vi "rqcBob Key Distribution (Low Level Example).vi"() -> ()   [LabVIEW 2018]
uses:
  FPGA/rqcBob/Custom Controls/rqcBob Trigger Type.ctl
  Custom Controls/rqcBob States.ctl
  Shared/Shared FPGA Lib/Shared Logic/Custom Controls/rqc Random Generator.parameters.ctl
  Shared/Shared FPGA Lib/Shared Logic/Custom Controls/rqc Random Generator.value type.ctl
  FPGA/rqcBob/Custom Controls/rqcBob Window Config.ctl
  FPGA/rqcBob/Custom Controls/rqcBob Modulator Config.ctl
  FPGA/rqcBob/Custom Controls/Pulse Train/rqcBob Pulse Train Config.ctl
  FPGA/rqcBob/Custom Controls/Pulse Train/rqcBob Pulse Train.Generation Mode.ctl
  FPGA/rqcBob/Custom Controls/Pulse Train/rqcBob Pulse Train.First Pulse Delay Mode.ctl
  Shared/Shared Host Lib/rqc ServiceNET/Custom Controls/rqc ServiceNET command.ctl
  Shared/Shared Host Lib/rqc ServiceNET/Bob/Custom Controls/rqcBob ServiceNET control.ctl
  <vilib>/FPGAPlugInAG/PCIe-7820R/niLvFpga_Open_PCIe-7820R.vi
  <vilib>/rvi/interface/common/dynamic/niFpgaDynamicAddResources.vi
  Low Level API/Configuration/Photon Detector/Set PD window/rqcBob Configure SPD Detection Window (2PD).vi
  Shared/Shared Host Lib/rqc ServiceNET/Bob/rqcBob Send Data/rqcBob ServiceNET Send Data U32.vi
  <vilib>/FPGAPlugInAG/Dynamic/niLvFpga_Close_Dynamic.vi
  <vilib>/rvi/interface/nirviOpenFPGA/nirviOpenFPGA.xnode
  FPGA Bitfiles/rqcBob (FPGA) 7820 v 4.0.0.lvbitx
  <vilib>/rvi/interface/nirviCloseFPGA/nirviCloseFPGA.xnode
panel:
  out "Bob's Key:":string="010100110101111110011011110000111111100101101001011100110010001011010011011001010000111101100001111011001111110010010110111100010001111011001000011001001101011000010111001010101110111010010000110011001101101100100101111100001111001011011110000010010101011001111010111001111100111110100100111011110001110101001100010011010001011011101010101000100011010101011010010001111110100010011010011001101101101000001100010110011001101001010101011000110010101100111101110101110011110100101100100001100100001101100001110010011000001101111001111110101101001010000110011100000011111101100010010100111000101011100110111010011100100000110000100110111101100000011011010011110000111011110111001101110001101011100111000010001001011000101100001110011001000100110101110010100000011011000001100111000101000100001110001001001011101100101101111000011101000111001110111000000101101000101011110101001101000001001000010011001010000011111111010010010001111011111001110001010100000010001000000101000000100101011010110100010111110111011110001100101010110010011101001010001100100000110000001111110101000001010000110001000011101110100110001000001100010101001000"
  in  "Modulator shift":fxp<+,4,4>=2.0
  in  "Check D2":u8=6
  in  "Random\nOn/Off":bool=TRUE
  in  "Pi Voltage":u16=140
  in  "2-Random (Up)\n4-Random (Down)":bool
  in  "Train Number":u16=1000
  in  "Pulses in Train":u16=500
  in  "Train Period":u16=4000
  in  "Open window":u16=2530
  out "Key length (s)":i32=2253
  out "Incorrect Alice's data":bool
  out "Total pulses expected:":u32=500000
  in  "Data shift":u8=3
  out "Current States":dbl=13.0
  out "error out":errorcluster
  out "Connected to Alice":bool
  in  "Stop":bool
  in  "Check D1":u8=24
  in  "Port:":u16=5020
  in  "Alice's IP address":string="192.168.0.175"
  # "BOB"
  # "FPGA settings:"
  # "LAN settings:"
  # "Key distillation details:"
  # "Data exchange details:"
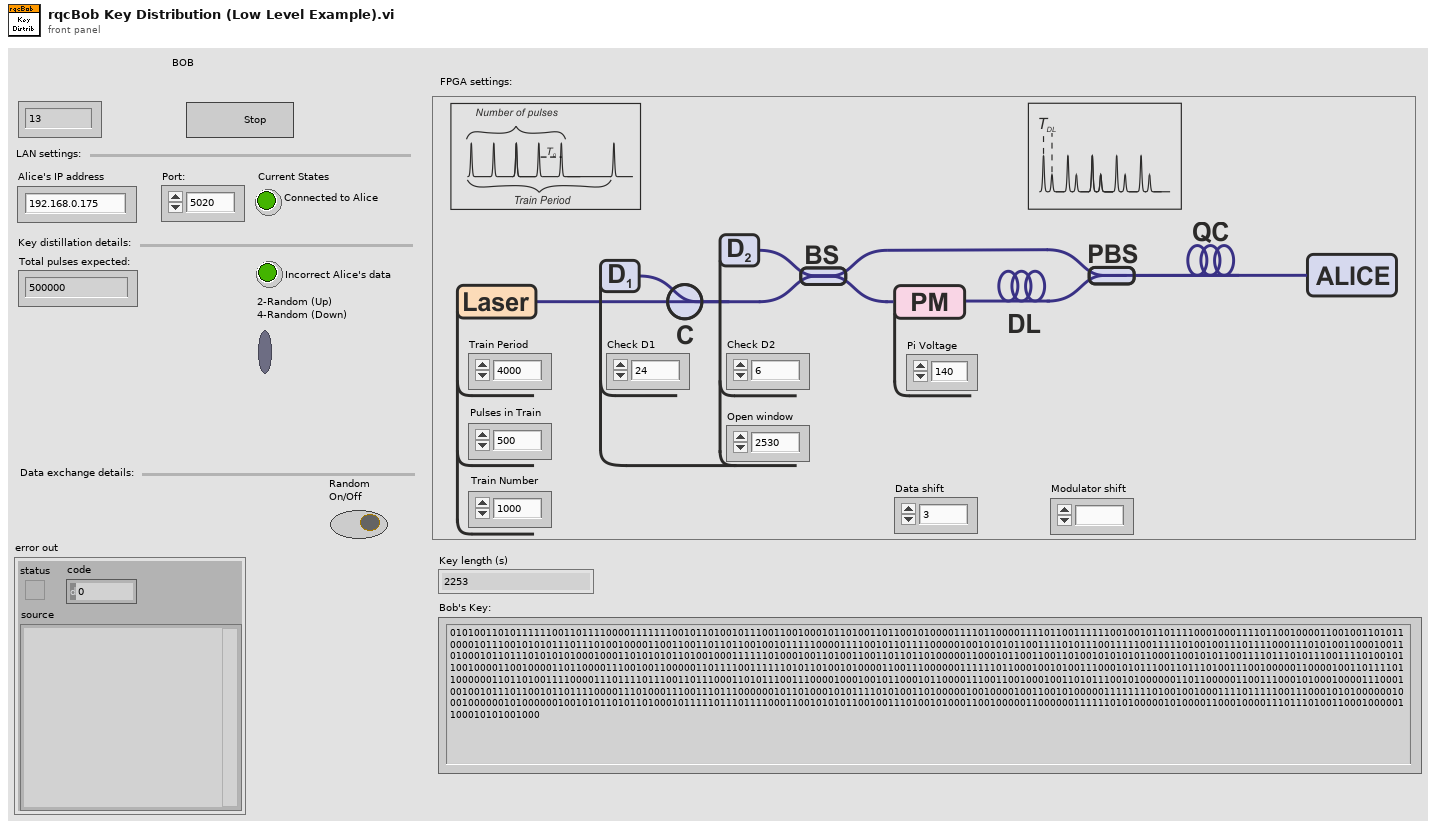
[diagram p1: front panel]
types:
  T1 = typedef "rqcBob States.ctl" = enum16{"HW.configure", "HW.sendTrigger", "HW.initiate", "HW.measure", "HW.stop", "NET.create", "NET.connect", "NET.sendCommand", "NET.readCommand", "NET.readData", "NET.close", "App.HandleEvent", "App.HandleError", "App.Stop"}
  T2 = typedef "rqcBob Trigger Type.ctl" = enum16{"software", "immediate", "DIO"}
  T3 = typedef "rqcBob Pulse Train Config.ctl" = cluster{"period":u16, "num of pulses":u16, "mode":T4, "num of trains":u16, "first pulse delay mode":T5, "first pulse delay":u16}
  T4 = typedef "rqcBob Pulse Train.Generation Mode.ctl" = enum8{"single train", "train sequence.single", "train sequence.wait for trigger", "continuous"}
  T5 = typedef "rqcBob Pulse Train.First Pulse Delay Mode.ctl" = enum8{"none", "every train", "first train"}
  T6 = typedef "rqcBob Modulator Config.ctl" = cluster{"modulator.start":u16, "modulator.stop":u16}
  T7 = typedef "rqcBob Window Config.ctl" = cluster{"window.open":u16, "window.close":u16}
  T8 = typedef "rqc Random Generator.parameters.ctl" = cluster{"value type":T9, "constant":u16, "num of levels":u16, "levels values":u16[]}
  T9 = typedef "rqc Random Generator.value type.ctl" = enum16{"random value", "constant"}
  T10 = typedef "rqc ServiceNET command.ctl" = enum8{"NONE", "READY", "START", "PING", "SEND KEY", "WRITE KEY", "WRITE AND SAVE KEY"}
  T11 = typedef "rqcBob ServiceNET control.ctl" = cluster{"connection ID":refnum<k5>, "connected?":bool, "Alice's IP address":string, "port":u16}
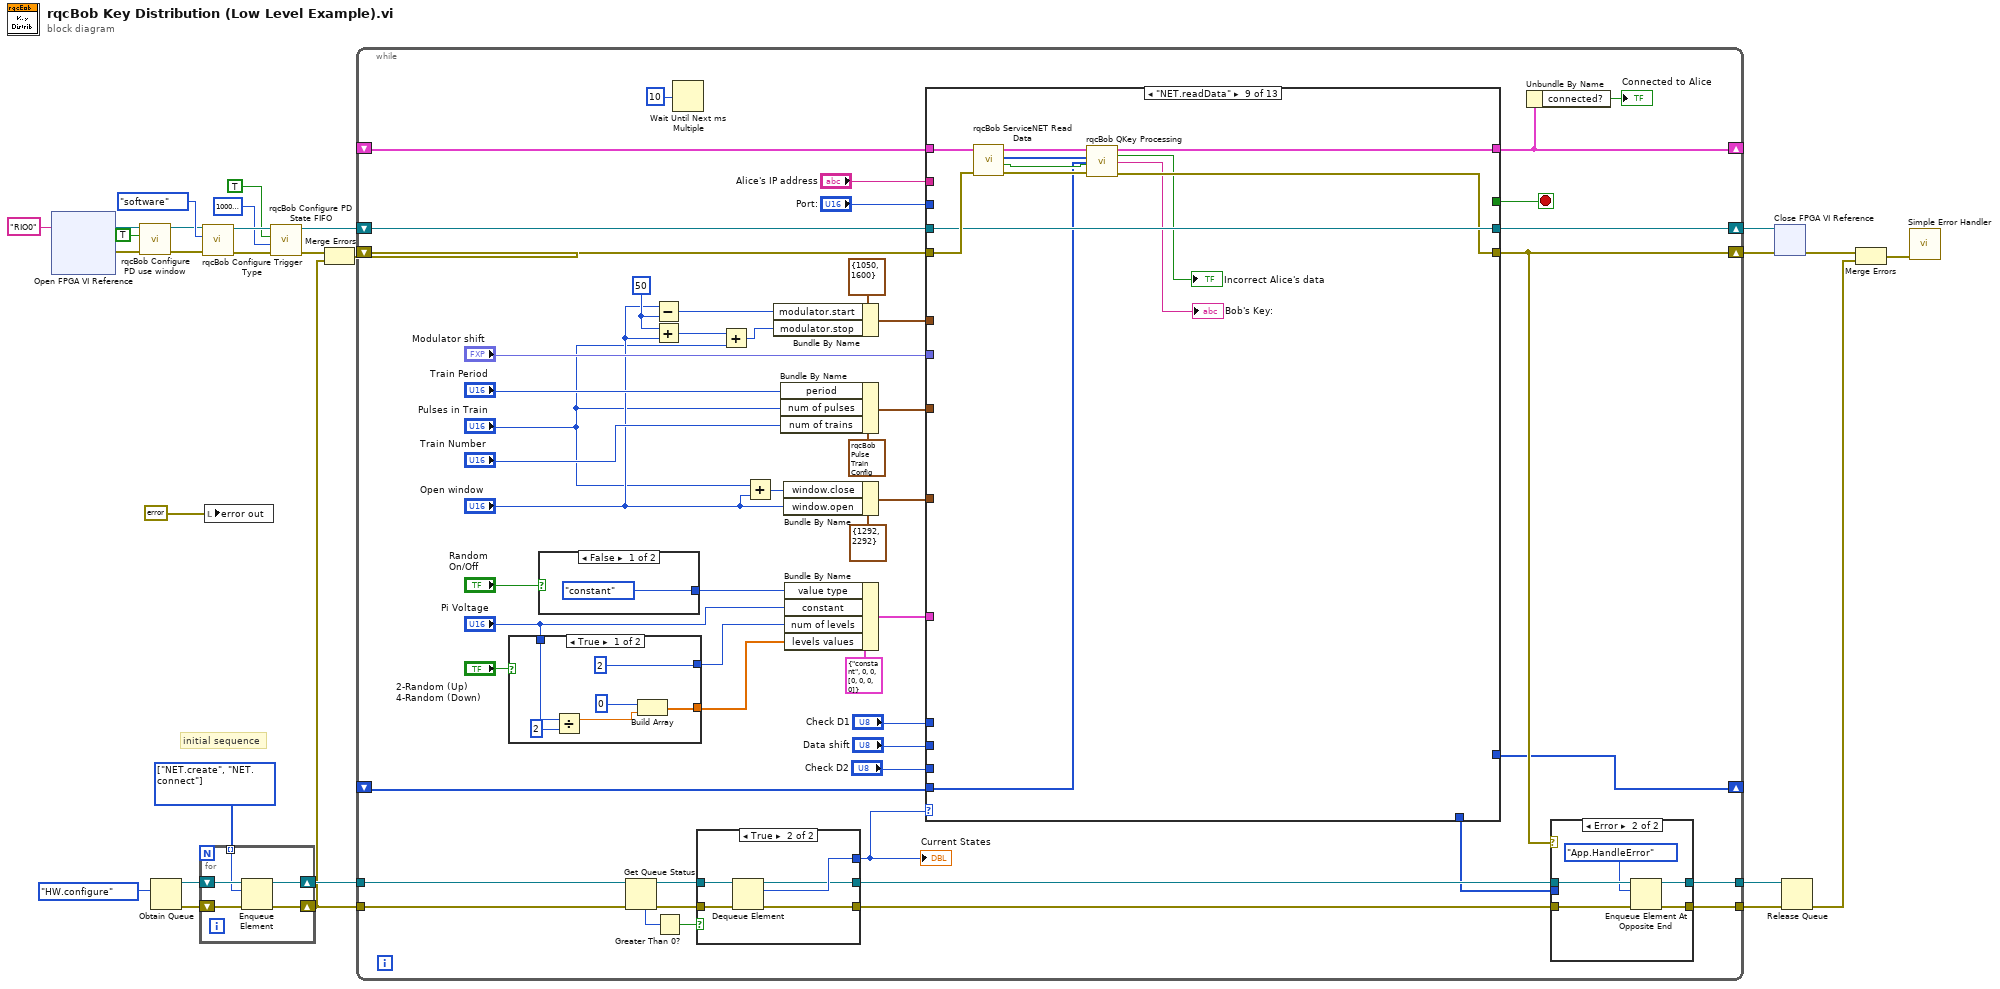
[diagram p0: block diagram]
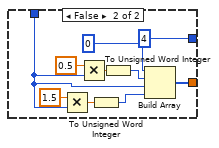
[diagram p2: hidden frame]
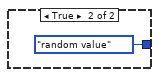
[diagram p3: hidden frame]
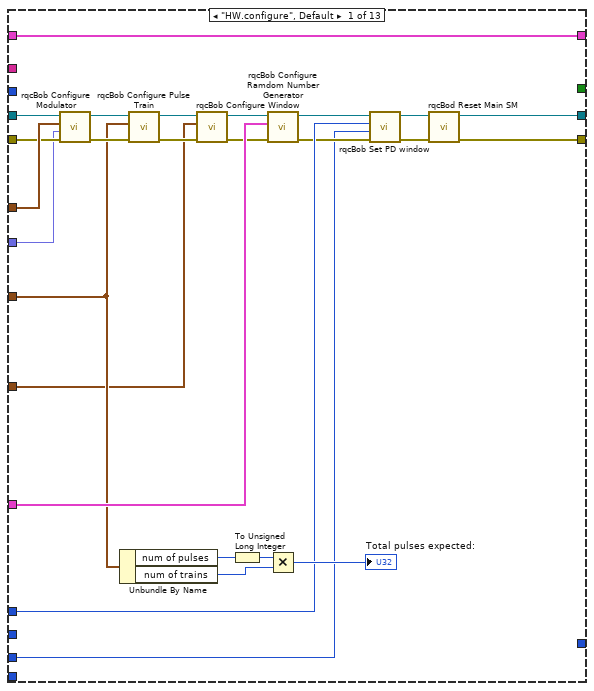
[diagram p4: hidden frame]
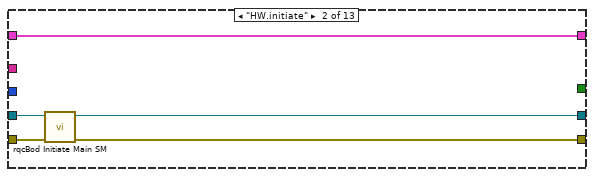
[diagram p5: hidden frame]
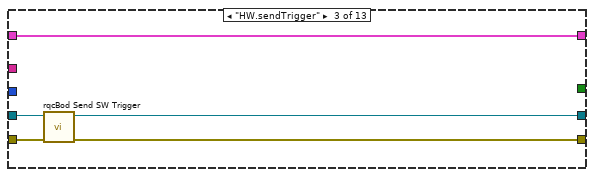
[diagram p6: hidden frame]
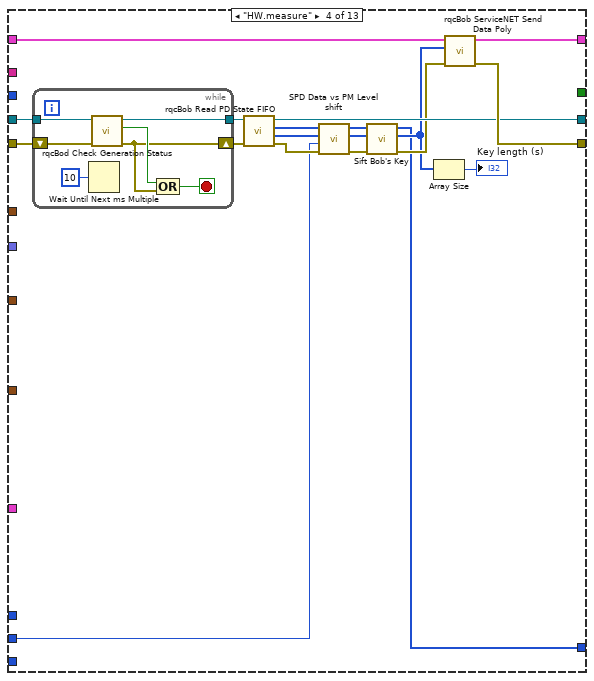
[diagram p7: hidden frame]
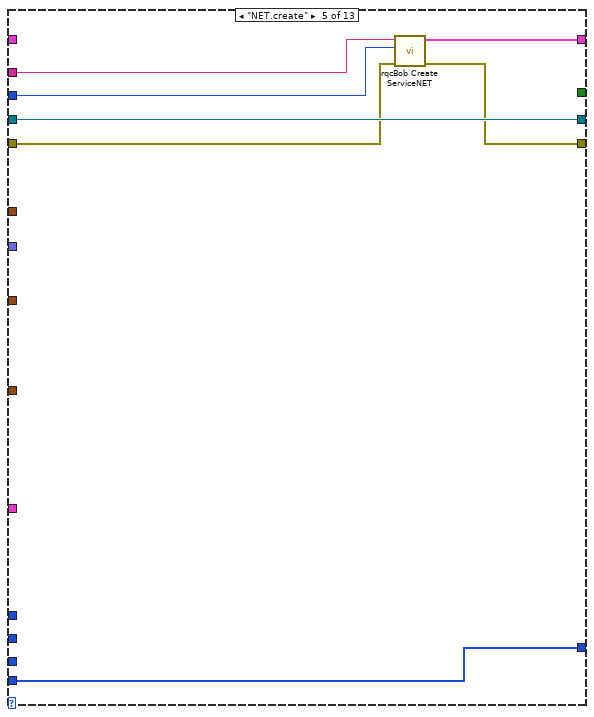
[diagram p8: hidden frame]
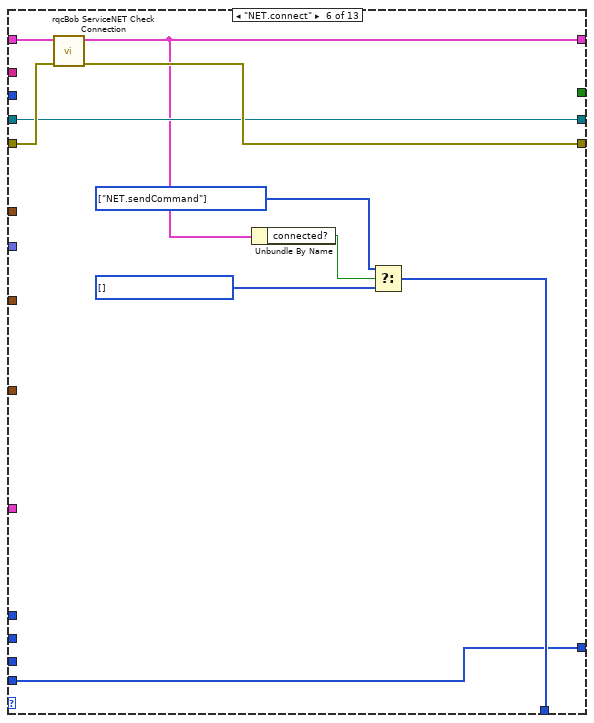
[diagram p9: hidden frame]
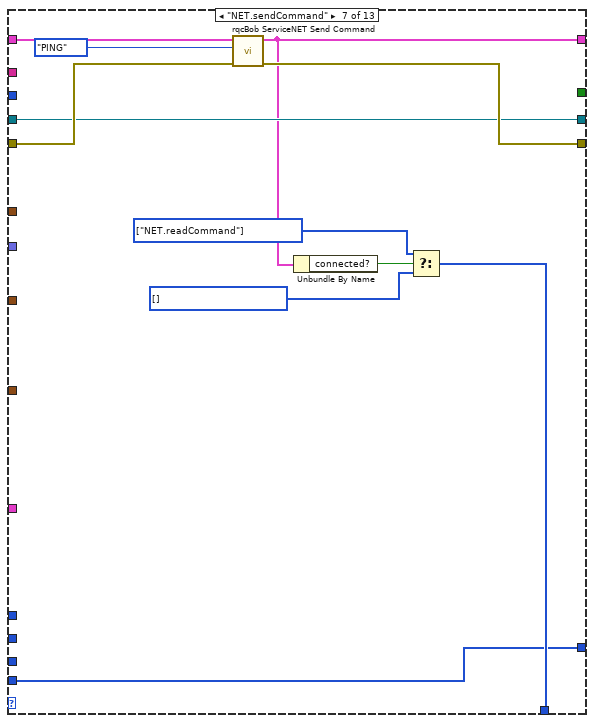
[diagram p10: hidden frame]
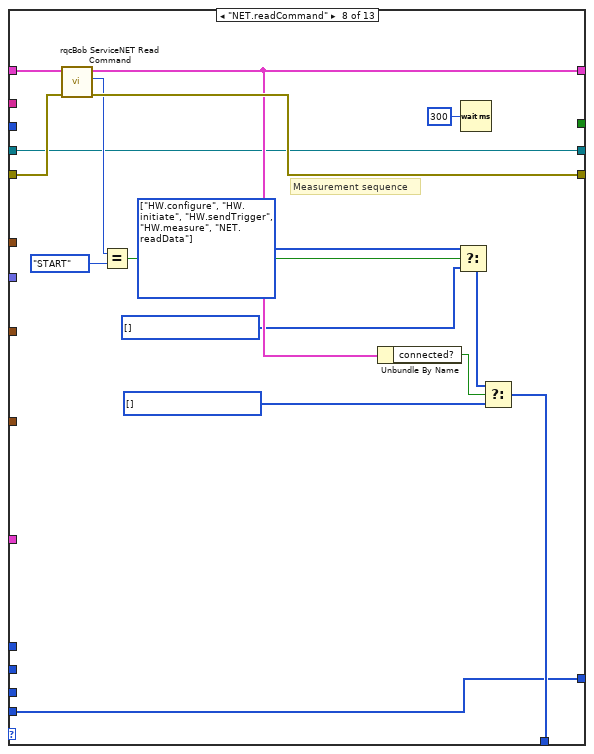
[diagram p11: hidden frame]
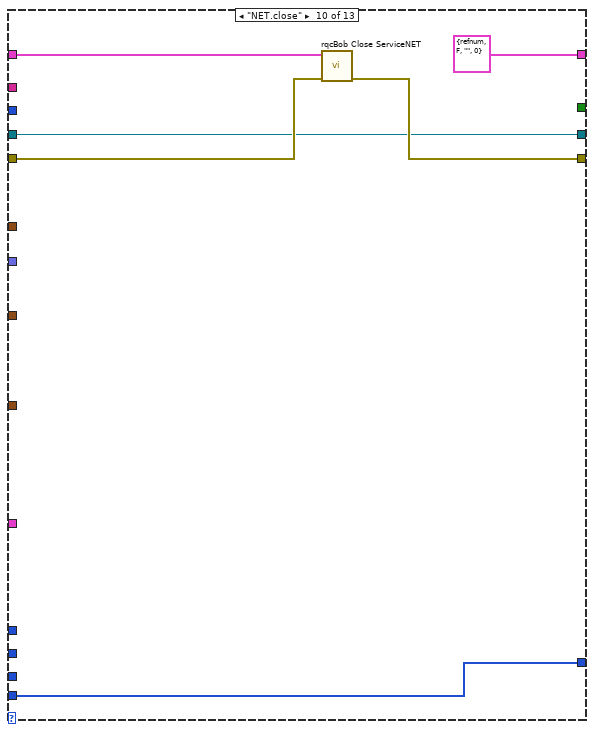
[diagram p12: hidden frame]
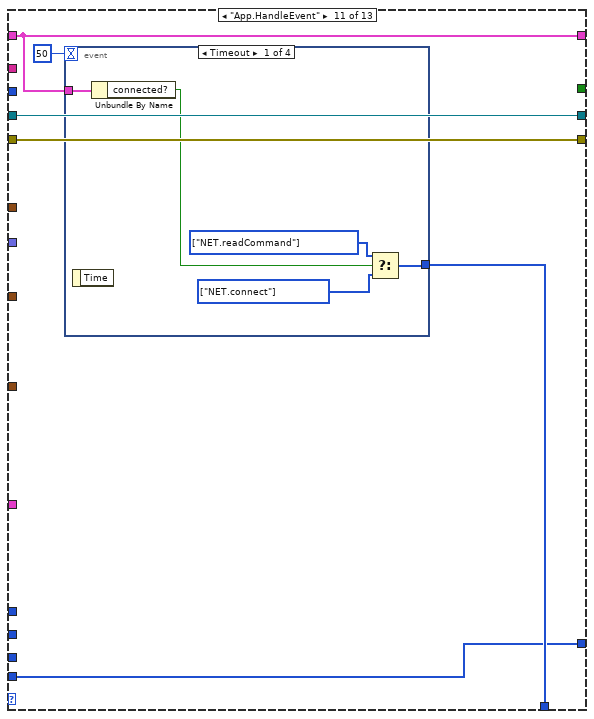
[diagram p13: hidden frame]
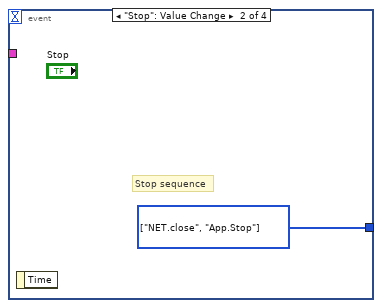
[diagram p14: hidden frame]
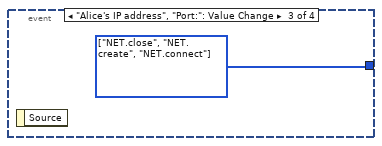
[diagram p15: hidden frame]
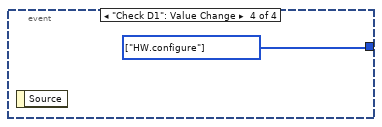
[diagram p16: hidden frame]
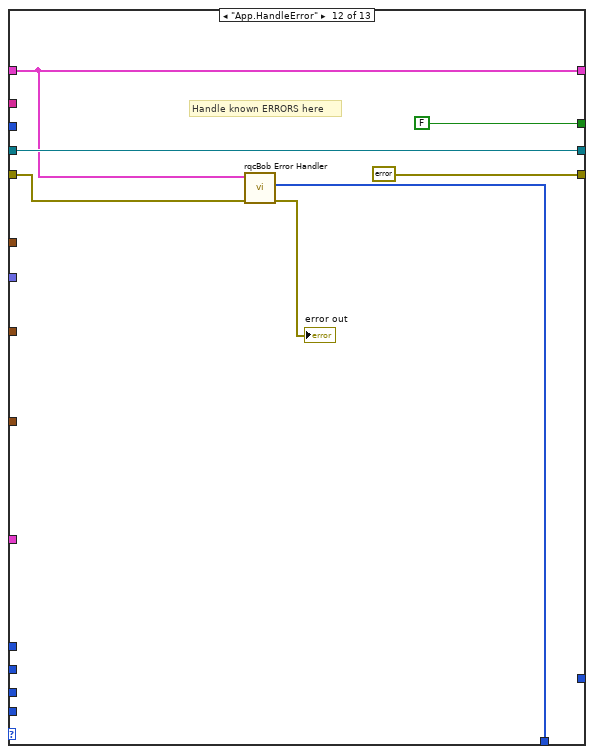
[diagram p17: hidden frame]
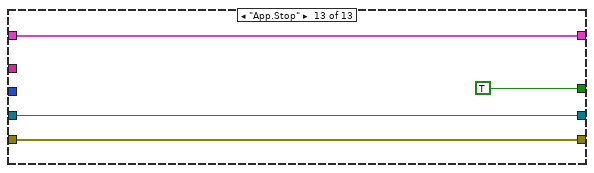
[diagram p18: hidden frame]
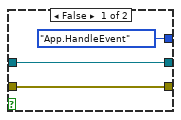
[diagram p19: hidden frame]
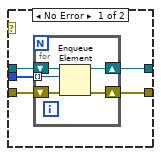
[diagram p20: hidden frame]
diagram:
  w21 = T1[] [enum."NET.create", enum."NET.connect"] items=["HW.configure", "HW.sendTrigger", "HW.initiate", "HW.measure", "HW.stop", "NET.create", "NET.connect", "NET.sendCommand", "NET.readCommand", "NET.readData", "NET.close", "App.HandleEvent", "App.HandleError", "App.Stop"]
  # "initial sequence"
  n1 = xnode "Open FPGA VI Reference"("resource name"="RIO0") -> ("FPGA VI Reference Out"=w5:refnum<k20>, "error out"=w3:errorcluster)  [unwired: 1 in]
  n2 = call "rqcBob Configure PD use window.vi"("error in"=w3, "PD.use window"=TRUE, "FPGA reference in"=w5) -> ("error out"=w2:errorcluster, "FPGA reference out"=w4:refnum<k20>)  [unwired: 7 in]
  n3 = Obtain Queue(element data type=rqcBob_States."HW.configure" ("rqcBob States")) -> (queue out=w26:refnum<queue>, error out=w25:errorcluster)  [unwired: 4 in, 1 out]
  n4 = for {
    tunnel: w21 -> [w29] mode=indexing
    shift-right: [w30] -> w23
    shift-left: w26 -> [w33]
    shift-right: [w31] -> w20
    shift-left: w25 -> [w32]
    n5 = Enqueue Element(queue=w33, element=w29, error in (no error)=w32) -> (queue out=w30:refnum<queue>, error out=w31:errorcluster)  [unwired: 1 in, 1 out]
  }
  n6 = call "rqcBob Configure Trigger Type.vi"("error in"=w2, "rqcBob Trigger Type"=rqcBob_Trigger_Type."software", "FPGA reference in"=w4) -> ("error out"=w8:errorcluster, "FPGA reference out"=w11:refnum<k20>)  [unwired: 7 in]
  n7 = local write "error out"(errorcluster {"status"=FALSE, "code"=0, "source"=""} ("error constant")) -> ()
  n8 = call "rqcBob Configure PD State FIFO.vi"("error in"=w8, "PD.state fifo depth"=u32 10000000 ("SPD.detect fifo depth"), "PD.state fifo write enable"=TRUE ("SPD.detect fifo write enable"), "FPGA reference in"=w11) -> ("error out"=w9:errorcluster, "FPGA reference out"=w10:refnum<k20>)  [unwired: 6 in]
  n9 = Merge Errors(w9, w20) -> (w24:errorcluster)
  n10 = while {
    shift-right: [w68] -> w19
    shift-left: w24 -> [w79]
    shift-right: [w69] -> w18
    shift-left: w10 -> [w66]
    tunnel: w23 -> [w77]
    tunnel: w20 -> [w76]
    tunnel: [w71] -> w17
    tunnel: [w70] -> w16
    shift-right: [w62] -> _
    shift-left: _ -> [w63]
    shift-right: [w58] -> _
    shift-left: _ -> [w57]
    stop <- w67 stop-if-true
    w49 = 50
    n11 = case shown="True" "2-Random (Up)\n4-Random (Down)" {
      tunnel: [w91 w92] -> w41
      tunnel: [u16 2 ("pm.DAC num of levels") u16 4 ("pm.DAC num of levels")] -> w40
      tunnel: "Pi Voltage" -> [w88 w93]
      frame True {
        n12 = Divide(x=w88, y=u16 2) -> (x/y=w87:dbl)
        n13 = Build Array(u16 0, w87) -> (w91:dbl[])
      }
      frame False {
        n14 = Multiply(x=1.5, y=w93) -> (x*y=w98:dbl)
        n15 = Multiply(x=0.5, y=w93) -> (x*y=w100:dbl)
        n16 = To Unsigned Word Integer(number=w98) -> (unsigned 16bit integer=w95:u16)
        n17 = To Unsigned Word Integer(number=w100) -> (unsigned 16bit integer=w96:u16)
        n18 = Build Array(u16 0, w96, w93, w95) -> (w92:u16[])
      }
    }
    n19 = case shown="False" "Random\nOn/Off" {
      tunnel: [rqc_Random_Generator.value_type."constant" ("value type") rqc_Random_Generator.value_type."random value" ("value type")] -> w42
      frame False {
      }
      frame True {
      }
    }
    n20 = Get Queue Status(queue=w77, error in (no error)=w76) -> (queue out=w73:refnum<queue>, error out=w72:errorcluster, # elements in queue=w75:i32)  [unwired: 1 in, 5 out]
    n21 = Subtract(x="Open window", y=w49) -> (x-y=w46:i32)
    n22 = Add(x=w49, y="Open window") -> (x+y=w45:i32)
    n23 = Greater Than 0?(x=w75) -> (x > 0?=w74:bool)
    n24 = Wait Until Next ms Multiple(millisecond multiple=u32 10) -> ()  [unwired: 1 out]
    n25 = case shown="True" w74 {
      tunnel: w73 -> [w253 w260]
      tunnel: w72 -> [w254 w259]
      tunnel: [rqcBob_States."App.HandleEvent" ("rqcBob States") w258] -> w82
      tunnel: [w253 w257] -> w81
      tunnel: [w254 w256] -> w78
      frame False {
      }
      frame True {
        n26 = Dequeue Element(queue=w260, error in (no error)=w259) -> (queue out=w257:refnum<queue>, element=w258:T1, error out=w256:errorcluster)  [unwired: 1 in, 1 out]
      }
    }
    "Current States" <- w82
    n27 = Add(x=w45, y="Pulses in Train") -> (x+y=w44:i32)
    n28 = Add(x="Pulses in Train", y="Open window") -> (x+y=w37:u16)
    n29 = Bundle By Name(cluster=T6 {"modulator.start"=1050, "modulator.stop"=1600} ("modulator.config"), "modulator.start"=w46, "modulator.stop"=w44) -> (w47:T6)
    n30 = Bundle By Name(cluster=T3 {"period"=4000, "num of pulses"=1000, "mode"=enum."train sequence.single", "num of trains"=1000, "first pulse delay mode"=enum."every train", "first pulse delay"=55} ("train.configuration"), "period"="Train Period", "num of pulses"="Pulses in Train", "num of trains"="Train Number") -> (w55:T3)
    n31 = Bundle By Name(cluster=T7 {"window.open"=1292, "window.close"=2292} ("window.config"), "window.close"=w37, "window.open"="Open window") -> (w56:T7)
    n32 = Bundle By Name(cluster=T8 {"value type"=enum."constant", "constant"=0, "num of levels"=0, "levels values"=[0, 0, 0, 0]} ("rqcBob rndGen.parameters"), "value type"=w42, "constant"="Pi Voltage", "num of levels"=w40, "levels values"=w41) -> (w53:T8)
    n33 = case shown="\"NET.readData\"" w82 {
      tunnel: w47 -> [w129 _ _ _ _ _ _ _ _ _ _ _ _]
      tunnel: w55 -> [w112 _ _ _ _ _ _ _ _ _ _ _ _]
      tunnel: w56 -> [w105 _ _ _ _ _ _ _ _ _ _ _ _]
      tunnel: w53 -> [w116 _ _ _ _ _ _ _ _ _ _ _ _]
      tunnel: "Check D1" -> [w119 _ _ _ _ _ _ _ _ _ _ _ _]
      tunnel: [w125 w131 w136 w154 w167 w180 w191 w207 w212 w224 w231 errorcluster {"status"=FALSE, "code"=0, "source"=""} ("error constant") w250] -> w68
      tunnel: w79 -> [w128 w133 w138 w157 w168 w181 w192 w208 w220 w225 w231 w245 w250]
      tunnel: [_ _ _ _ _ w174 w184 w203 _ _ w230 w244 _] -> w80
      tunnel: [w126 w132 w137 w151 w172 w179 w190 w196 w219 w223 w232 w247 w251] -> w69
      tunnel: [_ _ _ _ _ _ _ _ _ _ _ FALSE TRUE] -> w67
      tunnel: w66 -> [w127 w134 w139 w158 w172 w179 w190 w196 w219 w223 w232 w247 w251]
      tunnel: "Alice's IP address" -> [_ _ _ _ w171 _ _ _ _ _ _ _ _]
      tunnel: "Port:" -> [_ _ _ _ w170 _ _ _ _ _ _ _ _]
      tunnel: [w124 w130 w135 w156 w169 w178 w188 w204 w217 T11 {"connection ID"=refnum, "connected?"=FALSE, "Alice's IP address"="", "port"=0} ("rqcBob ServiceNET control") w229 w246 w249] -> w62
      tunnel: w63 -> [w124 w130 w135 w155 _ w182 w193 w209 w221 w227 w229 w246 w249]
      tunnel: "Data shift" -> [_ _ _ w145 _ _ _ _ _ _ _ _ _]
      tunnel: [_ _ _ w140 w166 w173 w183 w195 _ w222 w228 _ _] -> w58
      tunnel: w57 -> [_ _ _ _ w166 w173 w183 w195 w214 w222 w228 _ _]
      tunnel: "Modulator shift" -> [w115 _ _ _ _ _ _ _ _ _ _ _ _]
      tunnel: "Check D2" -> [w104 _ _ _ _ _ _ _ _ _ _ _ _]
      frame "HW.configure", Default {
        n34 = call "rqcBob Configure Modulator.vi"("error in"=w128, "modulator.clock delay"=w115, "modulator.config"=w129, "FPGA reference in"=w127) -> ("error out"=w113:errorcluster, "FPGA reference out"=w114:refnum<k20>)  [unwired: 6 in]
        n35 = Unbundle By Name(w112) -> ("num of pulses"=w122:u16, "num of trains"=w121:u16)
        n36 = call "rqcBob Configure Pulse Train.vi"("error in"=w113, "train.configuration"=w112, "FPGA reference in"=w114) -> ("error out"=w109:errorcluster, "FPGA reference out"=w110:refnum<k20>)  [unwired: 6 in, 1 out]
        n37 = call "rqcBob Configure Window.vi"("error in"=w109, "window.config"=w105, "FPGA reference in"=w110) -> ("error out"=w108:errorcluster, "FPGA reference out"=w111:refnum<k20>)  [unwired: 7 in]
        n38 = To Unsigned Long Integer(number=w122) -> (unsigned 32bit integer=w120:u32)
        n39 = call "rqcBob Configure Ramdom Number Generator.vi"("error in"=w108, "rqcBob rndGen.parameters"=w116, "FPGA reference in"=w111) -> ("error out"=w117:errorcluster, "FPGA reference out"=w118:refnum<k20>)  [unwired: 7 in]
        n40 = Multiply(x=w120, y=w121) -> (x*y=→"Total pulses expected:":u32)
        n41 = call-poly "rqcBob Set PD window.vi"("error in"=w117, "PD2.detection window"=w104, "PD1.detection window"=w119, "FPGA reference in"=w118) -> ("error out"=w107:errorcluster, "FPGA reference out"=w106:refnum<k20>)  [unwired: 6 in]
        n42 = call "rqcBod Reset Main SM.vi"("error in"=w107, "FPGA reference in"=w106) -> ("error out"=w125:errorcluster, "FPGA reference out"=w126:refnum<k20>)  [unwired: 8 in]
      }
      frame "HW.initiate" {
        n43 = call "rqcBod Initiate Main SM.vi"("error in"=w133, "FPGA reference in"=w134) -> ("error out"=w131:errorcluster, "FPGA reference out"=w132:refnum<k20>)  [unwired: 8 in]
      }
      frame "HW.sendTrigger" {
        n44 = call "rqcBod Send SW Trigger.vi"("error in"=w138, "FPGA reference in"=w139) -> ("error out"=w136:errorcluster, "FPGA reference out"=w137:refnum<k20>)  [unwired: 8 in]
      }
      frame "HW.measure" {
        n45 = while {
          tunnel: w158 -> [w165]
          shift-right: [w159] -> w152
          shift-left: w157 -> [w164]
          tunnel: [w161] -> w153
          stop <- w160 stop-if-true
          n46 = Wait Until Next ms Multiple(millisecond multiple=u32 10) -> ()  [unwired: 1 out]
          n47 = call "rqcBod Check Generation Status.vi"("error in"=w164, "FPGA reference in"=w165) -> ("error out"=w159:errorcluster, "generation.done"=w162:bool, "FPGA reference out"=w161:refnum<k20>)  [unwired: 7 in]
          n48 = Compound Arithmetic op=OR(w162, w159) -> (w160:bool)
        }
        n49 = call "rqcBob Read PD State FIFO.vi"("error in"=w152, "FPGA reference in"=w153) -> ("error out"=w147:errorcluster, "PM Level"=w143:u8[], "SPD Number"=w144:u8[], "FPGA reference out"=w151:refnum<k20>)  [unwired: 6 in]
        n50 = call "SPD Data vs PM Level shift.vi"("error in"=w147, "Data shift"=w145, "PM Level in"=w143, "SPD Number in"=w144) -> ("error out"=w150:errorcluster, "PM Level out"=w148:u8[], "SPD Number out"=w149:u8[])  [unwired: 5 in]
        n51 = call "Sift Bob's Key.vi"("error in"=w150, "PM Level in"=w148, "SPD Number in"=w149) -> ("error out"=w146:errorcluster, "Sifted Bob's data"=w141:u32[], "Raw Bob's data"=w140:u8[])  [unwired: 6 in]
        n52 = Array Size(array=w141) -> (size(s)=→"Key length (s)":i32)
        n53 = call-poly "rqcBob ServiceNET Send Data Poly.vi"("error in"=w146, "Data"=w141, "rqcBob ServiceNET in"=w155) -> ("error out"=w154:errorcluster, "rqcBob ServiceNET out"=w156:T11)  [unwired: 7 in]
      }
      frame "NET.create" {
        n54 = call "rqcBob Create ServiceNET.vi"("error in"=w168, "port"=w170, "Alice's IP address"=w171) -> ("error out"=w167:errorcluster, "rqcBob ServiceNET control"=w169:T11)  [unwired: 7 in]
      }
      frame "NET.connect" {
        w175 = T1[] [] items=["HW.configure", "HW.sendTrigger", "HW.initiate", "HW.measure", "HW.stop", "NET.create", "NET.connect", "NET.sendCommand", "NET.readCommand", "NET.readData", "NET.close", "App.HandleEvent", "App.HandleError", "App.Stop"] ("f")
        w177 = T1[] [enum."NET.sendCommand"] items=["HW.configure", "HW.sendTrigger", "HW.initiate", "HW.measure", "HW.stop", "NET.create", "NET.connect", "NET.sendCommand", "NET.readCommand", "NET.readData", "NET.close", "App.HandleEvent", "App.HandleError", "App.Stop"]
        n55 = call "rqcBob ServiceNET Check Connection.vi"("error in"=w181, "rqcBob ServiceNET in"=w182) -> ("error out"=w180:errorcluster, "rqcBob ServiceNET out"=w178:T11)  [unwired: 8 in]
        n56 = Unbundle By Name(w178) -> ("connected?"=w176:bool)
        n57 = Select(t=w177, s=w176, f=w175) -> (s? t:f=w174:T1[])
      }
      frame "NET.sendCommand" {
        w185 = T1[] [] items=["HW.configure", "HW.sendTrigger", "HW.initiate", "HW.measure", "HW.stop", "NET.create", "NET.connect", "NET.sendCommand", "NET.readCommand", "NET.readData", "NET.close", "App.HandleEvent", "App.HandleError", "App.Stop"] ("f")
        w186 = T1[] [enum."NET.readCommand"] items=["HW.configure", "HW.sendTrigger", "HW.initiate", "HW.measure", "HW.stop", "NET.create", "NET.connect", "NET.sendCommand", "NET.readCommand", "NET.readData", "NET.close", "App.HandleEvent", "App.HandleError", "App.Stop"] ("f")
        n58 = call "rqcBob ServiceNET Send Command.vi"("error in"=w192, "command"=rqc_ServiceNET_command."PING", "rqcBob ServiceNET in"=w193) -> ("error out"=w191:errorcluster, "rqcBob ServiceNET out"=w188:T11)  [unwired: 7 in]
        n59 = Unbundle By Name(w188) -> ("connected?"=w187:bool)
        n60 = Select(t=w186, s=w187, f=w185) -> (s? t:f=w184:T1[])
      }
      frame "NET.readCommand" {
        w198 = T1[] [] items=["HW.configure", "HW.sendTrigger", "HW.initiate", "HW.measure", "HW.stop", "NET.create", "NET.connect", "NET.sendCommand", "NET.readCommand", "NET.readData", "NET.close", "App.HandleEvent", "App.HandleError", "App.Stop"] ("f")
        w205 = T1[] [] items=["HW.configure", "HW.sendTrigger", "HW.initiate", "HW.measure", "HW.stop", "NET.create", "NET.connect", "NET.sendCommand", "NET.readCommand", "NET.readData", "NET.close", "App.HandleEvent", "App.HandleError", "App.Stop"] ("f")
        w199 = T1[] [enum."HW.configure", enum."HW.initiate", enum."HW.sendTrigger", enum."HW.measure", enum."NET.readData"] items=["HW.configure", "HW.sendTrigger", "HW.initiate", "HW.measure", "HW.stop", "NET.create", "NET.connect", "NET.sendCommand", "NET.readCommand", "NET.readData", "NET.close", "App.HandleEvent", "App.HandleError", "App.Stop"] ("f")
        # "Measurement sequence"
        n61 = call "rqcBob ServiceNET Read Command.vi"("error in"=w208, "rqcBob ServiceNET in"=w209) -> ("error out"=w207:errorcluster, "command"=w202:T10, "rqcBob ServiceNET out"=w204:T11)  [unwired: 6 in, 1 out]
        n62 = Equal?(x=w202, y=rqc_ServiceNET_command."START") -> (x = y?=w200:bool)
        n63 = Unbundle By Name(w204) -> ("connected?"=w206:bool)
        n64 = Select(t=w199, s=w200, f=w198) -> (s? t:f=w197:T1[])
        n65 = Wait (ms)(milliseconds to wait=u32 300) -> ()  [unwired: 1 out]
        n66 = Select(t=w197, s=w206, f=w205) -> (s? t:f=w203:T1[])
      }
      frame "NET.readData" {
        n67 = call "rqcBob ServiceNET Read Data.vi"("error in"=w220, "rqcBob ServiceNET in"=w221) -> ("error out"=w216:errorcluster, "data valid"=w215:bool, "Data"=w213:u32[], "rqcBob ServiceNET out"=w218:T11)  [unwired: 6 in]
        n68 = call "rqcBob QKey Processing.vi"("rqcBob ServiceNET in"=w218, "Correct indices"=w213, "Raw Bob's data"=w214, "data valid"=w215, "error in"=w216) -> ("rqcBob ServiceNET out"=w217:T11, "Incorrect Alice's data"=→"Incorrect Alice's data":bool, "Bob's Key:"=→"Bob's Key:":string, "error out"=w212:errorcluster)  [unwired: 7 in]
      }
      frame "NET.close" {
        n69 = call "rqcBob Close ServiceNET.vi"("error in"=w225, "rqcBob ServiceNET control"=w227) -> ("error out"=w224:errorcluster)  [unwired: 9 in]
      }
      frame "App.HandleEvent" {
        n70 = event shown="[0] Timeout" {
          selector: _ -> [_ _ _ _]
          dyn-events: _ -> [_ _ _ _]
          timeout: 50 -> [_ _ _ _]
          tunnel: [w237 w239 w240 w241] -> w230
          tunnel: w229 -> [w238 _ _ _]
          event Timeout {
            w234 = T1[] [enum."NET.connect"] items=["HW.configure", "HW.sendTrigger", "HW.initiate", "HW.measure", "HW.stop", "NET.create", "NET.connect", "NET.sendCommand", "NET.readCommand", "NET.readData", "NET.close", "App.HandleEvent", "App.HandleError", "App.Stop"]
            w235 = T1[] [enum."NET.readCommand"] items=["HW.configure", "HW.sendTrigger", "HW.initiate", "HW.measure", "HW.stop", "NET.create", "NET.connect", "NET.sendCommand", "NET.readCommand", "NET.readData", "NET.close", "App.HandleEvent", "App.HandleError", "App.Stop"]
            n71 = event-data() -> ()  [unwired: 1 in, 1 out]
            n72 = Unbundle By Name(w238) -> ("connected?"=w236:bool)
            n73 = Select(t=w235, s=w236, f=w234) -> (s? t:f=w237:T1[])
          }
          event "Stop": Value Change {
            w239 = T1[] [enum."NET.close", enum."App.Stop"] items=["HW.configure", "HW.sendTrigger", "HW.initiate", "HW.measure", "HW.stop", "NET.create", "NET.connect", "NET.sendCommand", "NET.readCommand", "NET.readData", "NET.close", "App.HandleEvent", "App.HandleError", "App.Stop"]
            # "Stop sequence"
            n74 = event-data() -> ()  [unwired: 1 in, 1 out]
          }
          event "Alice's IP address", "Port:": Value Change {
            w240 = T1[] [enum."NET.close", enum."NET.create", enum."NET.connect"] items=["HW.configure", "HW.sendTrigger", "HW.initiate", "HW.measure", "HW.stop", "NET.create", "NET.connect", "NET.sendCommand", "NET.readCommand", "NET.readData", "NET.close", "App.HandleEvent", "App.HandleError", "App.Stop"]
            n75 = event-data() -> ()  [unwired: 1 in, 1 out]
          }
          event "Check D1": Value Change {
            w241 = T1[] [enum."HW.configure"] items=["HW.configure", "HW.sendTrigger", "HW.initiate", "HW.measure", "HW.stop", "NET.create", "NET.connect", "NET.sendCommand", "NET.readCommand", "NET.readData", "NET.close", "App.HandleEvent", "App.HandleError", "App.Stop"]
            n76 = event-data() -> ()  [unwired: 1 in, 1 out]
          }
        }
      }
      frame "App.HandleError" {
        # "Handle known ERRORS here"
        n77 = call "rqcBob Error Handler.vi"("error in (no error)"=w245, "rqcBob ServiceNET control"=w246) -> ("error out"=→"error out":errorcluster, "error sequence"=w244:T1[])  [unwired: 8 in]
      }
      frame "App.Stop" {
      }
    }
    n78 = Unbundle By Name(w62) -> ("connected?"=→"Connected to Alice":bool)
    n79 = case shown="Error" w68 {
      tunnel: w81 -> [w265 w275]
      tunnel: w80 -> [w262 _]
      tunnel: w78 -> [w261 w274]
      tunnel: [w264 w272] -> w71
      tunnel: [w263 w271] -> w70
      frame No Error {
        n80 = for {
          tunnel: w262 -> [w269] mode=indexing
          shift-right: [w267] -> w263
          shift-left: w261 -> [w268]
          shift-right: [w266] -> w264
          shift-left: w265 -> [w270]
          n81 = Enqueue Element(queue=w270, element=w269, error in (no error)=w268) -> (queue out=w266:refnum<queue>, error out=w267:errorcluster)  [unwired: 1 in, 1 out]
        }
      }
      frame Error {
        n82 = Enqueue Element At Opposite End(queue=w275, element=rqcBob_States."App.HandleError", error in (no error)=w274) -> (queue out=w272:refnum<queue>, error out=w271:errorcluster)  [unwired: 1 in, 1 out]
      }
    }
  }
  n83 = xnode "Close FPGA VI Reference"("FPGA VI Reference In"=w18, "error in"=w19) -> ("error out"=w15:errorcluster)
  n84 = Release Queue(queue=w17, error in (no error)=w16) -> (error out=w14:errorcluster)  [unwired: 1 in, 2 out]
  n85 = Merge Errors(w15, w14) -> (w13:errorcluster)
  n86 = call <vilib>:"Simple Error Handler.vi"("error in (no error)"=w13) -> ()  [unwired: 4 in, 5 out]
